vi "GetStepName.vi"(8 "error in":errorcluster, 11 "StepRun in":refnum<class "StepRun.lvclass">) -> (0 "error out":errorcluster, 2 "StepName":string, 3 "StepRun out":refnum<class "StepRun.lvclass">)   [LabVIEW 2021, in "ProligentXMLGenerator.lvlib" / "StepRun.lvclass"]
doc: "Defines the step name for the current step run.\n\nThis value is restricted to 255 chars."
uses:
  StepRun.lvclass
  StepRun.lvclass/StepRun.ctl
  Base/NonEmptyString_255/NonEmptyString_255.lvclass
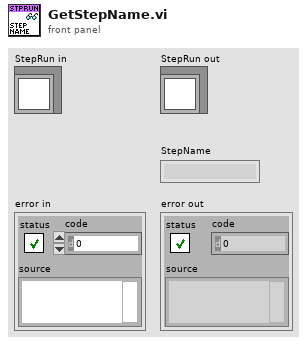
[diagram p1: front panel]
types:
  T1 = typedef "ProligentXMLGenerator.lvlib/StepRun.lvclass/Data.ctl" = cluster{"Name":string, "Measures":refnum<class "Measure.lvclass">[], "FailureReferences":refnum<class "FailureReference.lvclass">[], "Characteristics":refnum<class "Characteristic.lvclass">[], "Documents":refnum<class "Document.lvclass">[], "CustomData":refnum<class "CustomData.lvclass">, "StepExecutionStatus":refnum<class "ExecutionStatus.lvclass">, "StepRunId":refnum<class "Guid.lvclass">, "StepName":refnum<class "NonEmptyString_255.lvclass">, "StartDate":refnum<class "DateTime.lvclass">, "EndDate":refnum<class "DateTime.lvclass">, "TimeZoneInfoId":string}
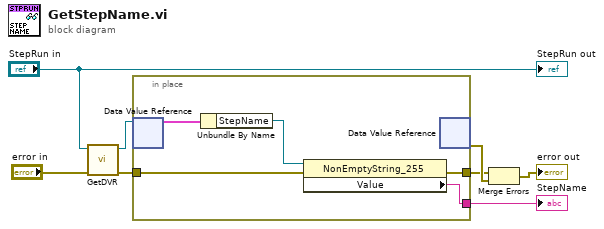
[diagram p0: block diagram]
diagram:
  n1 = call "GetDVR.vi"("error in"="error in", "StepRun"="StepRun in") -> ("error out"=w2:errorcluster, "DVRReference"=w7:refnum<data-value>)  [unwired: 8 in]
  n2 = in-place "In Place Element Structure" {
    in-place-border: [w10] -> w6
    in-place-border: w2 -> [w11]
    in-place-border: [w9] -> w1
    n3 = in-place-dvr #1(w7) -> (w13:T1)  [unwired: 1 out]
    n4 = Unbundle By Name(w13) -> ("StepName"=w12:refnum<class "NonEmptyString_255.lvclass">)
    n5 = property on="Property Node" class="NonEmptyString_255"(reference=w12, error in=w11) -> (error out=w9:errorcluster, "Value"=w10:string)  [unwired: 1 out]
    n6 = in-place-dvr #1() -> (w8:errorcluster)  [unwired: 1 in, 1 out]
  }
  "StepName" <- w6
  n7 = Merge Errors(w1, w8) -> (→"error out":errorcluster)
  "StepRun out" <- "StepRun in"
